vi "Test Quartz Counter.vi"() -> ()   [LabVIEW 2011, in "Diamond Universal Driver.lvlib"]
uses:
  Diamond Universal Driver.lvlib
  Controls/dscqmmcmr.ctl
  Controls/QMM Gating Control.ctl
  Controls/counter source.ctl
  Controls/Output Control.ctl
  Controls/QMM ACTION.ctl
  Controls/board type.ctl
  Controls/dsccb.ctl
  Controls/dscBool.ctl
  constants.vi
panel:
  out "x-y":u16
  out "error out":errorcluster
  out "count":u16
  in  "Boolean":bool
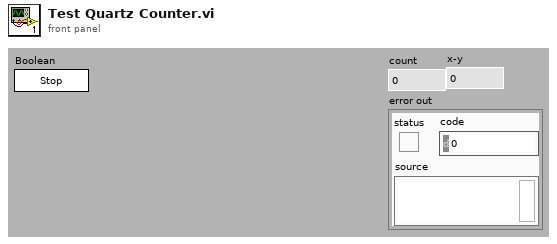
[diagram p1: front panel]
types:
  T1 = typedef "QMM ACTION.ctl" = enum8{"NONE", "ARM", "LOAD", "LOAD AND ARM", "DISARM AND SAVE", "SAVE", "DISARM"}
  T2 = typedef "dsccb.ctl" = cluster{"board type":T3, "board num":i16, "base addr":u16, "int level":u8, "RMM external trig":T4, "RMM external trig c3":T4, "EMM IOAdd":u16[], "EMM IOInterrupt":u16[], "clkfreq0":enum8{"10 MHz", "1 MHz"}, "clkfreq1":enum8{"10 MHz", "1 MHz"}, "clksel1":enum8{"Internal (clkfrq1)", "External"}, "address space":dbl, "DAC cfg":u8, "clck_freq":i32, "dma_level":u8, "int_lvl 1":u8, "int_lvl 2":u8, "int_lvl 3":u8, "fpga":u16, "smm_ad_res":u8, "RMM mode 16bit":T4, "RMM DAC 0_3 ext en":T4, "RMM DAC 4_7 ext en":T4}
  T3 = typedef "board type.ctl" = u8
  T4 = typedef "dscBool.ctl" = i32
  T5 = typedef "dscqmmcmr.ctl" = cluster{"counter":u8, "gating control":T6, "active source edge":enum8{"Rising", "Falling"}, "count source":T7, "special gate":enum8{"enable", "disable"}, "reload source":enum8{"Load register", "Load or hold register"}, "cycle":enum8{"one shot", "recycle"}, "count type":enum8{"binary", "BCD"}, "count direction":enum8{"down", "up"}, "output control":T8}
  T6 = typedef "Diamond Universal Driver.lvlib/QMM Gating Control.ctl" = enum8{"NO GATING", "ACTIVE HIGH TC NM1", "ACTIVE HIGH LEVEL GATE NP1", "ACTIVE HIGH LEVEL GATE NM1", "ACTIVE HIGH LEVEL GATE N", "ACTIVE LOW LEVEL GATE N", "ACTIVE HIGH EDGE GATE N", "ACTIVE LOW EDGE GATE N"}
  T7 = typedef "Diamond Universal Driver.lvlib/counter source.ctl" = enum8{"E1_TC_NM1", "SRC1", "SRC2", "SRC3", "SRC4", "SRC5", "GATE1", "GATE2", "GATE3", "GATE4", "GATE5", "F1_4MHZ", "F2_400KHZ", "F3_40KHZ", "F4_4KHZ", "F5_400HZ"}
  T8 = typedef "Diamond Universal Driver.lvlib/Output Control.ctl" = enum8{"INACTIVE OUTPUT LOW", "ACTIVE HIGH PULSE ON TC", "TOGGLE ON TC", "INACTIVE OUTPUT HIGH", "ACTIVE LOW PULSE ON TC"}
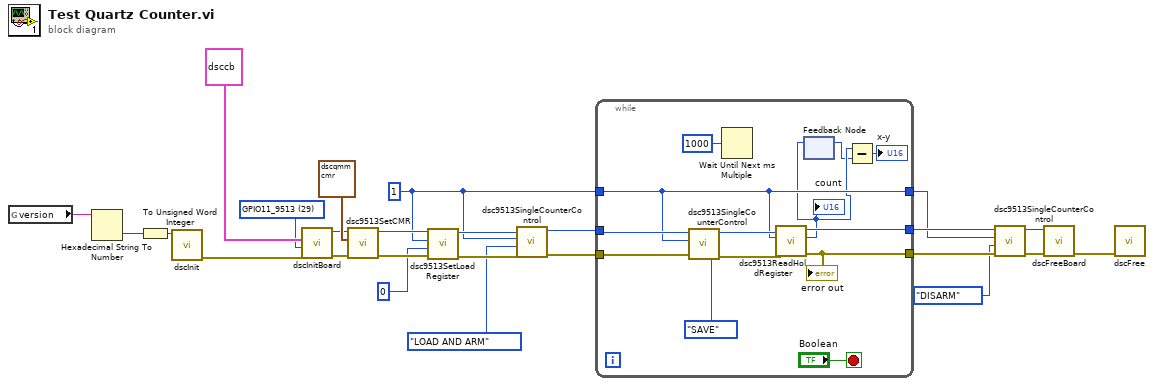
[diagram p0: block diagram]
diagram:
  w12 = T3 29 items=["DMM16"=0, "RMM"=1, "TMM"=2, "OPMM"=3, "DMM"=4, "SMM"=5, "GMM"=6, "QMM"=7, "ZMM"=8, "PMM"=9, "OMM"=10, "RMM416"=11, "DMM32AT"=12, "EMMDIO"=13, "RMM1612"=14, "DMMAT"=15, "DMM16AT"=16, "IR104"=17, "EMM8"=18, "PROM"=19, "HERCEBX"=20, "CPT"=21, "DMM48AT"=22, "OMMIO"=23, "DIO82C55"=24, "ATHENA"=25, "METIS"=26, "DMM32XAT"=27, "ELEKTRA"=28, "GPIO11_9513"=29, "GPIO11_DIO"=30, "GPIO21"=31, "PSD"=32, "ATHENAII"=33, "DMM32DXAT"=34, "HELIOS"=35, "NEPTUNE"=36, "TEST"=126, "RAW"=127, "DRVR"=255] ("board type")
  w16 = u8 1 ("counter")
  n1 = global read "constants.vi" "version"() -> (w3:string)
  n2 = Hexadecimal String To Number(string=w3) -> (number=w2:u32)  [unwired: 2 in, 1 out]
  n3 = To Unsigned Word Integer(number=w2) -> (unsigned 16bit integer=w1:u16)
  n4 = call "dscInit.vi"("versionIn"=w1) -> ("error out"=w14:errorcluster)  [unwired: 9 in, 1 out]
  n5 = call "dscInitBoard.vi"("error in"=w14, "board type"=w12, "DSCCB"=T2 {"board type"=29, "board num"=1, "base addr"=832, "int level"=0, "RMM external trig"=0, "RMM external trig c3"=0, "EMM IOAdd"=[], "EMM IOInterrupt"=[], "clkfreq0"=enum."10 MHz", "clkfreq1"=enum."10 MHz", "clksel1"=enum."Internal (clkfrq1)", "address space"=0.0, "DAC cfg"=0, "clck_freq"=0, "dma_level"=0, "int_lvl 1"=0, "int_lvl 2"=0, "int_lvl 3"=0, "fpga"=0, "smm_ad_res"=0, "RMM mode 16bit"=0, "RMM DAC 0_3 ext en"=0, "RMM DAC 4_7 ext en"=0}) -> ("error out"=w10:errorcluster, "boardHandleOut"=w11:i16)  [unwired: 6 in, 1 out]
  n6 = call "dsc9513SetCMR.vi"("error in"=w10, "cmr"=T5 {"counter"=1, "gating control"=enum."NO GATING", "active source edge"=enum."Rising", "count source"=enum."SRC1", "special gate"=enum."disable", "reload source"=enum."Load register", "cycle"=enum."recycle", "count type"=enum."binary", "count direction"=enum."up", "output control"=enum."INACTIVE OUTPUT LOW"}, "board"=w11) -> ("error out"=w23:errorcluster, "boardOut"=w24:i16)  [unwired: 7 in]
  n7 = call "dsc9513SetLoadRegister.vi"("error in"=w23, "value"=u16 0, "counter"=w16, "board"=w24) -> ("error out"=w20:errorcluster, "boardOut"=w21:i16)  [unwired: 6 in]
  n8 = call "dsc9513SingleCounterControl.vi"("error in"=w20, "action"=QMM_ACTION."LOAD AND ARM", "counter"=w16, "board"=w21) -> ("error out"=w17:errorcluster, "boardOut"=w18:i16)  [unwired: 5 in, 1 out]
  n9 = while {
    tunnel: w18 -> [w38]
    tunnel: w17 -> [w36]
    tunnel: w16 -> [w30]
    tunnel: [w32] -> w9
    tunnel: [w31] -> w8
    tunnel: [w30] -> w4
    stop <- "Boolean" stop-if-true
    n10 = call "dsc9513SingleCounterControl.vi"("error in"=w36, "action"=QMM_ACTION."SAVE", "counter"=w30, "board"=w38) -> ("error out"=w35:errorcluster, "boardOut"=w34:i16)  [unwired: 5 in, 1 out]
    n11 = Wait Until Next ms Multiple(millisecond multiple=u32 1000) -> ()  [unwired: 1 out]
    n12 = call "dsc9513ReadHoldRegister.vi"("error in"=w35, "counter"=w30, "board"=w34) -> ("error out"=w31:errorcluster, "counter_out"=w28:u8, "boardOut"=w32:i16)  [unwired: 5 in, 1 out]
    "count" <- w28
    "error out" <- w31
    n13 = feedback-in #1(w28) -> ()
    n14 = feedback #1() -> (w27:u8)  [unwired: 1 in]
    n15 = Subtract(x=w28, y=w27) -> (x-y=→"x-y":u8)
  }
  n16 = call "dsc9513SingleCounterControl.vi"("error in"=w8, "action"=QMM_ACTION."DISARM", "counter"=w4, "board"=w9) -> ("error out"=w6:errorcluster, "boardOut"=w7:i16)  [unwired: 5 in, 1 out]
  n17 = call "dscFreeBoard.vi"("error in"=w6, "boardIn"=w7) -> ("error out"=w15:errorcluster)  [unwired: 8 in, 1 out]
  n18 = call "dscFree.vi"("error in"=w15) -> ()  [unwired: 10 in, 1 out]
